vi "createDirectories.vi"(8 "error in (no error)":errorcluster, 10 "TimeStamp":string, 11 "FileNeologist in":refnum<class "FileNeologist.lvclass">) -> (0 "error out":errorcluster, 3 "FileNeologist out":refnum<class "FileNeologist.lvclass">)   [LabVIEW 2011, in "Tools.lvlib" / "Filing.lvlib" / "FileNeologist.lvclass"]
uses:
  FileNeologist.lvclass
  FileNeologist.lvclass/FileNeologist.ctl
  FileSystem/FileSystem.lvclass
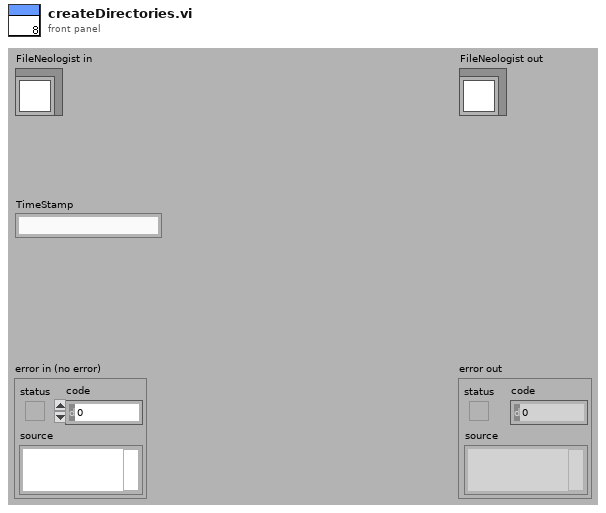
[diagram p1: front panel]
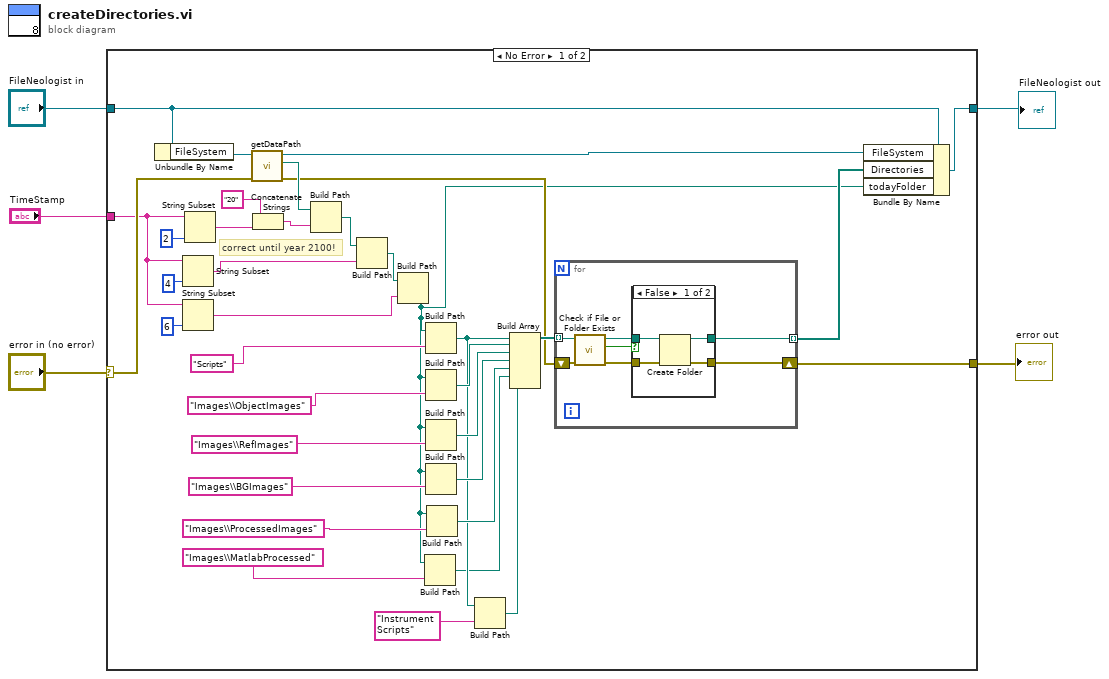
[diagram p0: block diagram]
diagram:
  n1 = case shown="No Error" "error in (no error)" {
    selector: "error in (no error)" -> [w40 w56]
    tunnel: [w22 w56] -> w4
    tunnel: [w19 w55] -> w2
    tunnel: "FileNeologist in" -> [w20 w55]
    tunnel: "TimeStamp" -> [w36 _]
    frame No Error {
      # "correct until year 2100!"
      n2 = Unbundle By Name(w20) -> ("FileSystem"=w41:refnum<class "FileSystem.lvclass">)
      n3 = String Subset(string=w36, length (rest)=4) -> (substring=w33:string)  [unwired: 1 in]
      n4 = String Subset(string=w36, length (rest)=6) -> (substring=w31:string)  [unwired: 1 in]
      n5 = String Subset(string=w36, length (rest)=2) -> (substring=w17:string)  [unwired: 1 in]
      n6 = call-dynamic "getDataPath.vi"("error in (no error)"=w40, "FileSystem.lvclass in"=w41) -> ("error out"=w23:errorcluster, "DataPath"=w35:path, "FileSystem.lvclass out"=w18:refnum<class "FileSystem.lvclass">)  [unwired: 7 in]
      n7 = Concatenate Strings("20", w17) -> (w15:string)
      n8 = Build Path(base path=w35, name or relative path=w15) -> (appended path=w34:path)
      n9 = Build Path(base path=w34, name or relative path=w33) -> (appended path=w32:path)
      n10 = Build Path(base path=w32, name or relative path=w31) -> (appended path=w9:path)
      n11 = Build Path(base path=w9, name or relative path="Images\\MatlabProcessed") -> (appended path=w7:path)
      n12 = Build Path(base path=w9, name or relative path="Scripts") -> (appended path=w11:path)
      n13 = Build Path(base path=w9, name or relative path="Images\\ObjectImages") -> (appended path=w28:path)
      n14 = Build Path(base path=w9, name or relative path="Images\\RefImages") -> (appended path=w27:path)
      n15 = Build Path(base path=w9, name or relative path="Images\\BGImages") -> (appended path=w26:path)
      n16 = Build Path(base path=w9, name or relative path="Images\\ProcessedImages") -> (appended path=w25:path)
      n17 = Build Path(base path=w11, name or relative path="Instrument Scripts") -> (appended path=w6:path)
      n18 = Build Array(w11, w28, w27, w26, w25, w7, w6) -> (w24:path[])
      n19 = for {
        tunnel: w24 -> [w45] mode=indexing
        shift-right: [w43] -> w22
        shift-left: w23 -> [w44]
        tunnel: [w42] -> w21 mode=indexing
        n20 = call <vilib>:"Check if File or Folder Exists.vi"("error in (no error)"=w44, "path"=w45) -> ("error out"=w46:errorcluster, "file or folder exists?"=w48:bool, "dup path"=w47:path)  [unwired: 7 in]
        n21 = case shown="False" w48 {
          tunnel: w47 -> [w52 w54]
          tunnel: [w49 w54] -> w42
          tunnel: w46 -> [w51 w53]
          tunnel: [w50 w53] -> w43
          frame False {
            n22 = Create Folder(path (use dialog)=w52, error in=w51) -> (created path=w49:path, error out=w50:errorcluster)  [unwired: 1 in, 1 out]
          }
          frame True {
          }
        }
      }
      n23 = Bundle By Name(cluster=w20, "FileSystem"=w18, "Directories"=w21, "todayFolder"=w9) -> (w19:refnum<class "FileNeologist.lvclass">)
    }
    frame Error {
    }
  }
  "error out" <- w4
  "FileNeologist out" <- w2
